vi "final_usrp_transceiver2.vi"() -> ()   [LabVIEW 2014]
uses:
  <vilib>/addons/Modulation/Analog/support/mod_Set Error Source.vi
  var_stop.vi
  <vilib>/addons/Modulation/Digital/Support/Common/Validators/mod_Generate Filter Coefficients Validate.vi
  <vilib>/addons/Modulation/Digital/General/subVIs/mod_Generate Filter Coefficients.vi
  <vilib>/measure/maspectr.llb/FFT Power Spectrum and PSD for 1 Chan (CDB).vi
  <vilib>/addons/Modulation/Digital/General/MT Apply Matched Filter (Generic).vi
  <vilib>/addons/Modulation/Digital/General/MT Align to Ideal Symbols (Generic).vi
  <instrlib>/niUSRP/niUSRP Fetch Rx Data (CDB Cluster).vi
  <instrlib>/niUSRP/niUSRP Write Tx Data (CDB Cluster).vi
  <vilib>/addons/Modulation/Digital/General/MT Apply Pulse Shaping Filter (Generic).vi
  <vilib>/addons/Modulation/niDMT.lvlib
  <vilib>/measure/NI_MAPro.lvlib
panel:
  in  "frame buffer size":i32=20
  in  "Stop":bool
  out "Frames Per Second":u32
  in  "energy threshold":dbl=-33.0 format="%#_13g"
  out "elements in frame buffer 2":i32
  out "elements in frame buffer":i32
  out "valid frames":i32
  out "elements in send buffer":i32
  in  "packet size":i32=12800
  in  "Quality (0-1000)":i32=100 caption="Quality (750)"
  out "size(s) 4":i32
  out "frame num":u32
  out "length":i32[](array[numeric])
  out "start index":i32[](array[numeric])
  out "Numeric":i32
  out "size(s) 3":i32
  out "# elements in queue 2":i32
  out "size(s) 2":i32
  out "size(s)":i32[](array[numeric])
  out "image":T1(plugin-control)
  in  "Transmit power (db)":dbl
  out "found?":bool
  out "# elements in queue":i32
  out "valid?":bool
  in  "Gray code?":bool=TRUE
  in  "Modulation":enum16{"PSK", "QAM"}(ring)
  out "packet len":u32
  in  "filter length (symbols)":i32=8
  in  "filter parameter":dbl=0.5 format="%.2f"
  in  "pulse shaping filter (none)":T2(ring)=enum."Raised Cosine"
  in  "M-PSK (4)":i32=4 caption="M-ARY"
  in  "samples per symbol (16)":i32=4
  out "packet bits length":i32
  in  "number of samples":i64=40000
  out "RX coerced gain":dbl format="%#_6f"
  out "RX coerced carrier frequency":dbl=915000000.0 format="%#_6p"
  out "RX coerced IQ rate":dbl=4000000.0 format="%#_6p"
  in  "RX active antenna":string="RX2"
  in  "RX gain":dbl format="%#_6f"
  in  "RX device names":refnum<k15>="192.168.10.2"
  out "TX coerced gain":dbl format="%#_6f"
  out "TX coerced carrier frequency":dbl=915000000.0 format="%#_6p"
  out "coerced IQ rate":dbl=4000000.0 format="%#_6p"
  in  "TX device names":refnum<k15>="192.168.10.2"
  in  "TX gain":dbl format="%#_6f"
  in  "carrier frequency":dbl=915000000.0 format="%#_6p"
  in  "IQ rate":dbl=800000.0 format="%#_6p"
  in  "stop":bool
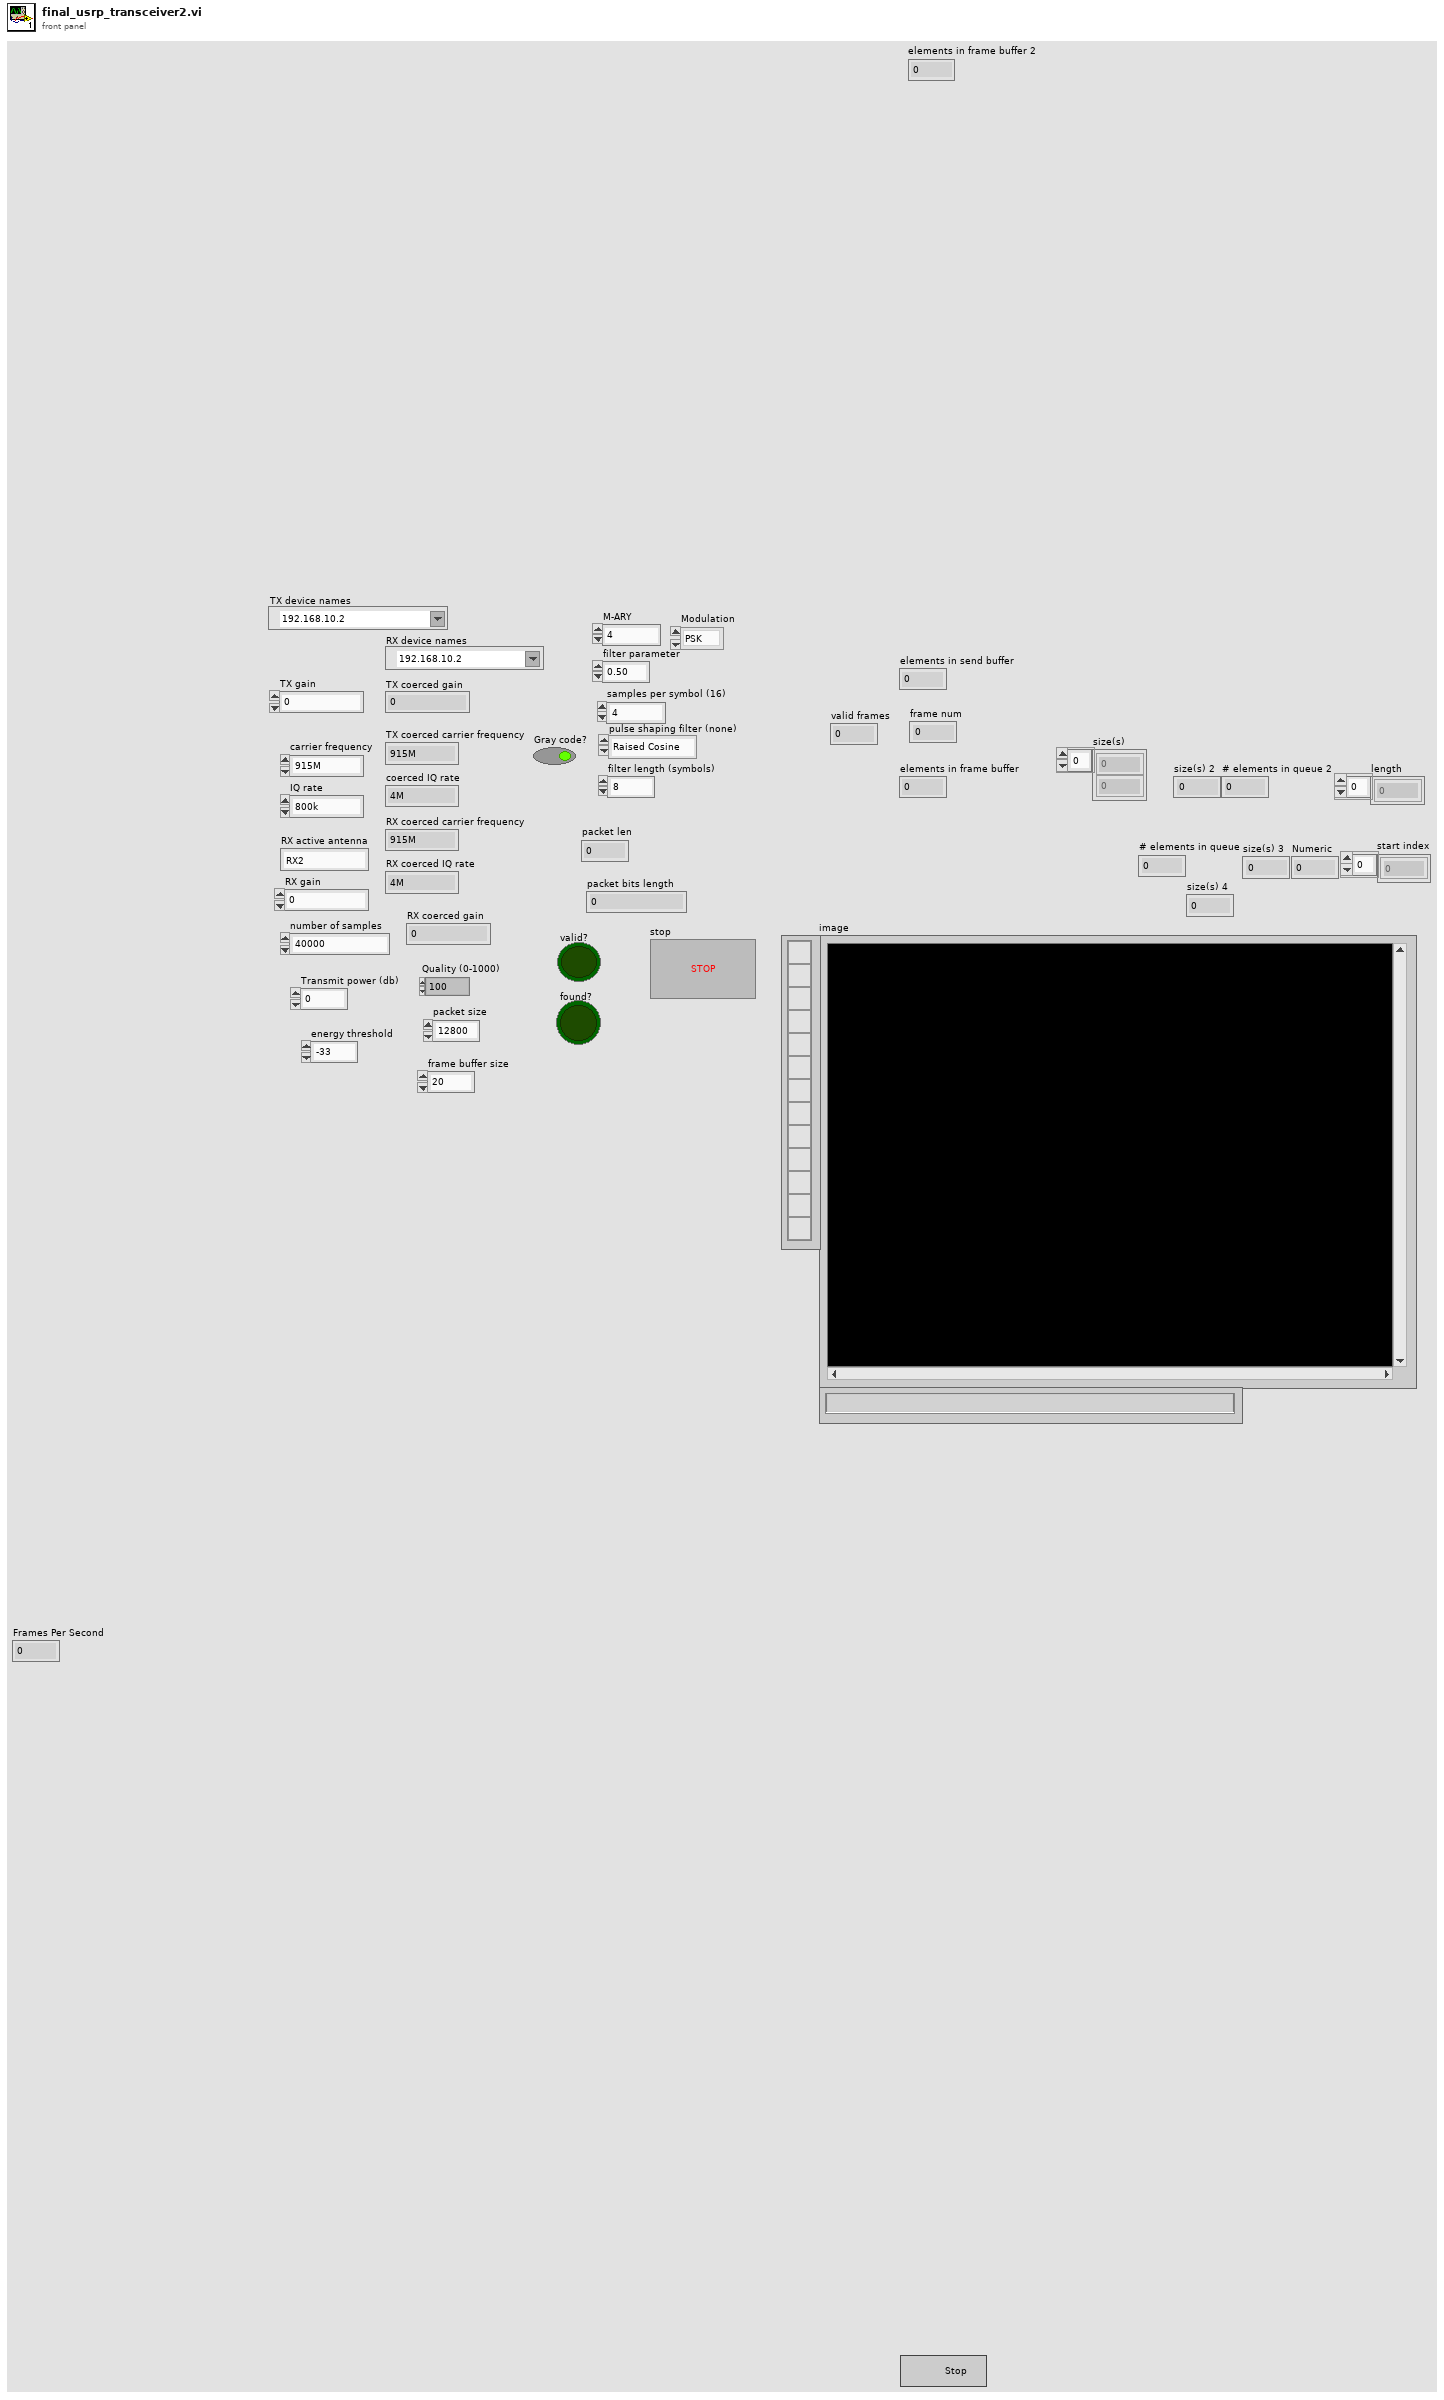
[diagram p1: front panel]
types:
  T1 = typedef "IMAQ Image.ctl" = refnum<image>
  T2 = enum16{"none", "Raised Cosine", "Root Raised Cos", "Gaussian"}
  T3 = enum16{"FSK", "PSK", "QAM", "MSK", "PAM", "ASK", "CPM"}
  T4 = cluster{"samples per symbol (16)":i32, "symbol map":cdb[], "index map":u32[]}
  T5 = cluster{"samples per symbol (16)":i32, "symbol map":cdb[], i32[]}
  T6 = typedef "IMAQ AVI2 Refnum.ctl" = refnum<k20>
  T7 = typedef "Image Type" = u32
  T8 = cluster{"Width":u32, "Height":u32, "Frames Per Second":u32, "Codec":string, "Has Data":bool}
  T9 = typedef "Semaphore RefNum" = refnum<k1>
  T10 = typedef "niAMT.lvlib/Complex Data Waveform.ctl" = cluster{"t0":dbl, "dt":dbl, "Y":cdb[]}
  T11 = typedef "imagedata.ctl" = cluster{"image type":i32, "image depth":i32, "image":u8[], "mask":u8[], "colors":u32[], "Rectangle":cluster{"left":i16, "top":i16, "right":i16, "bottom":i16}}
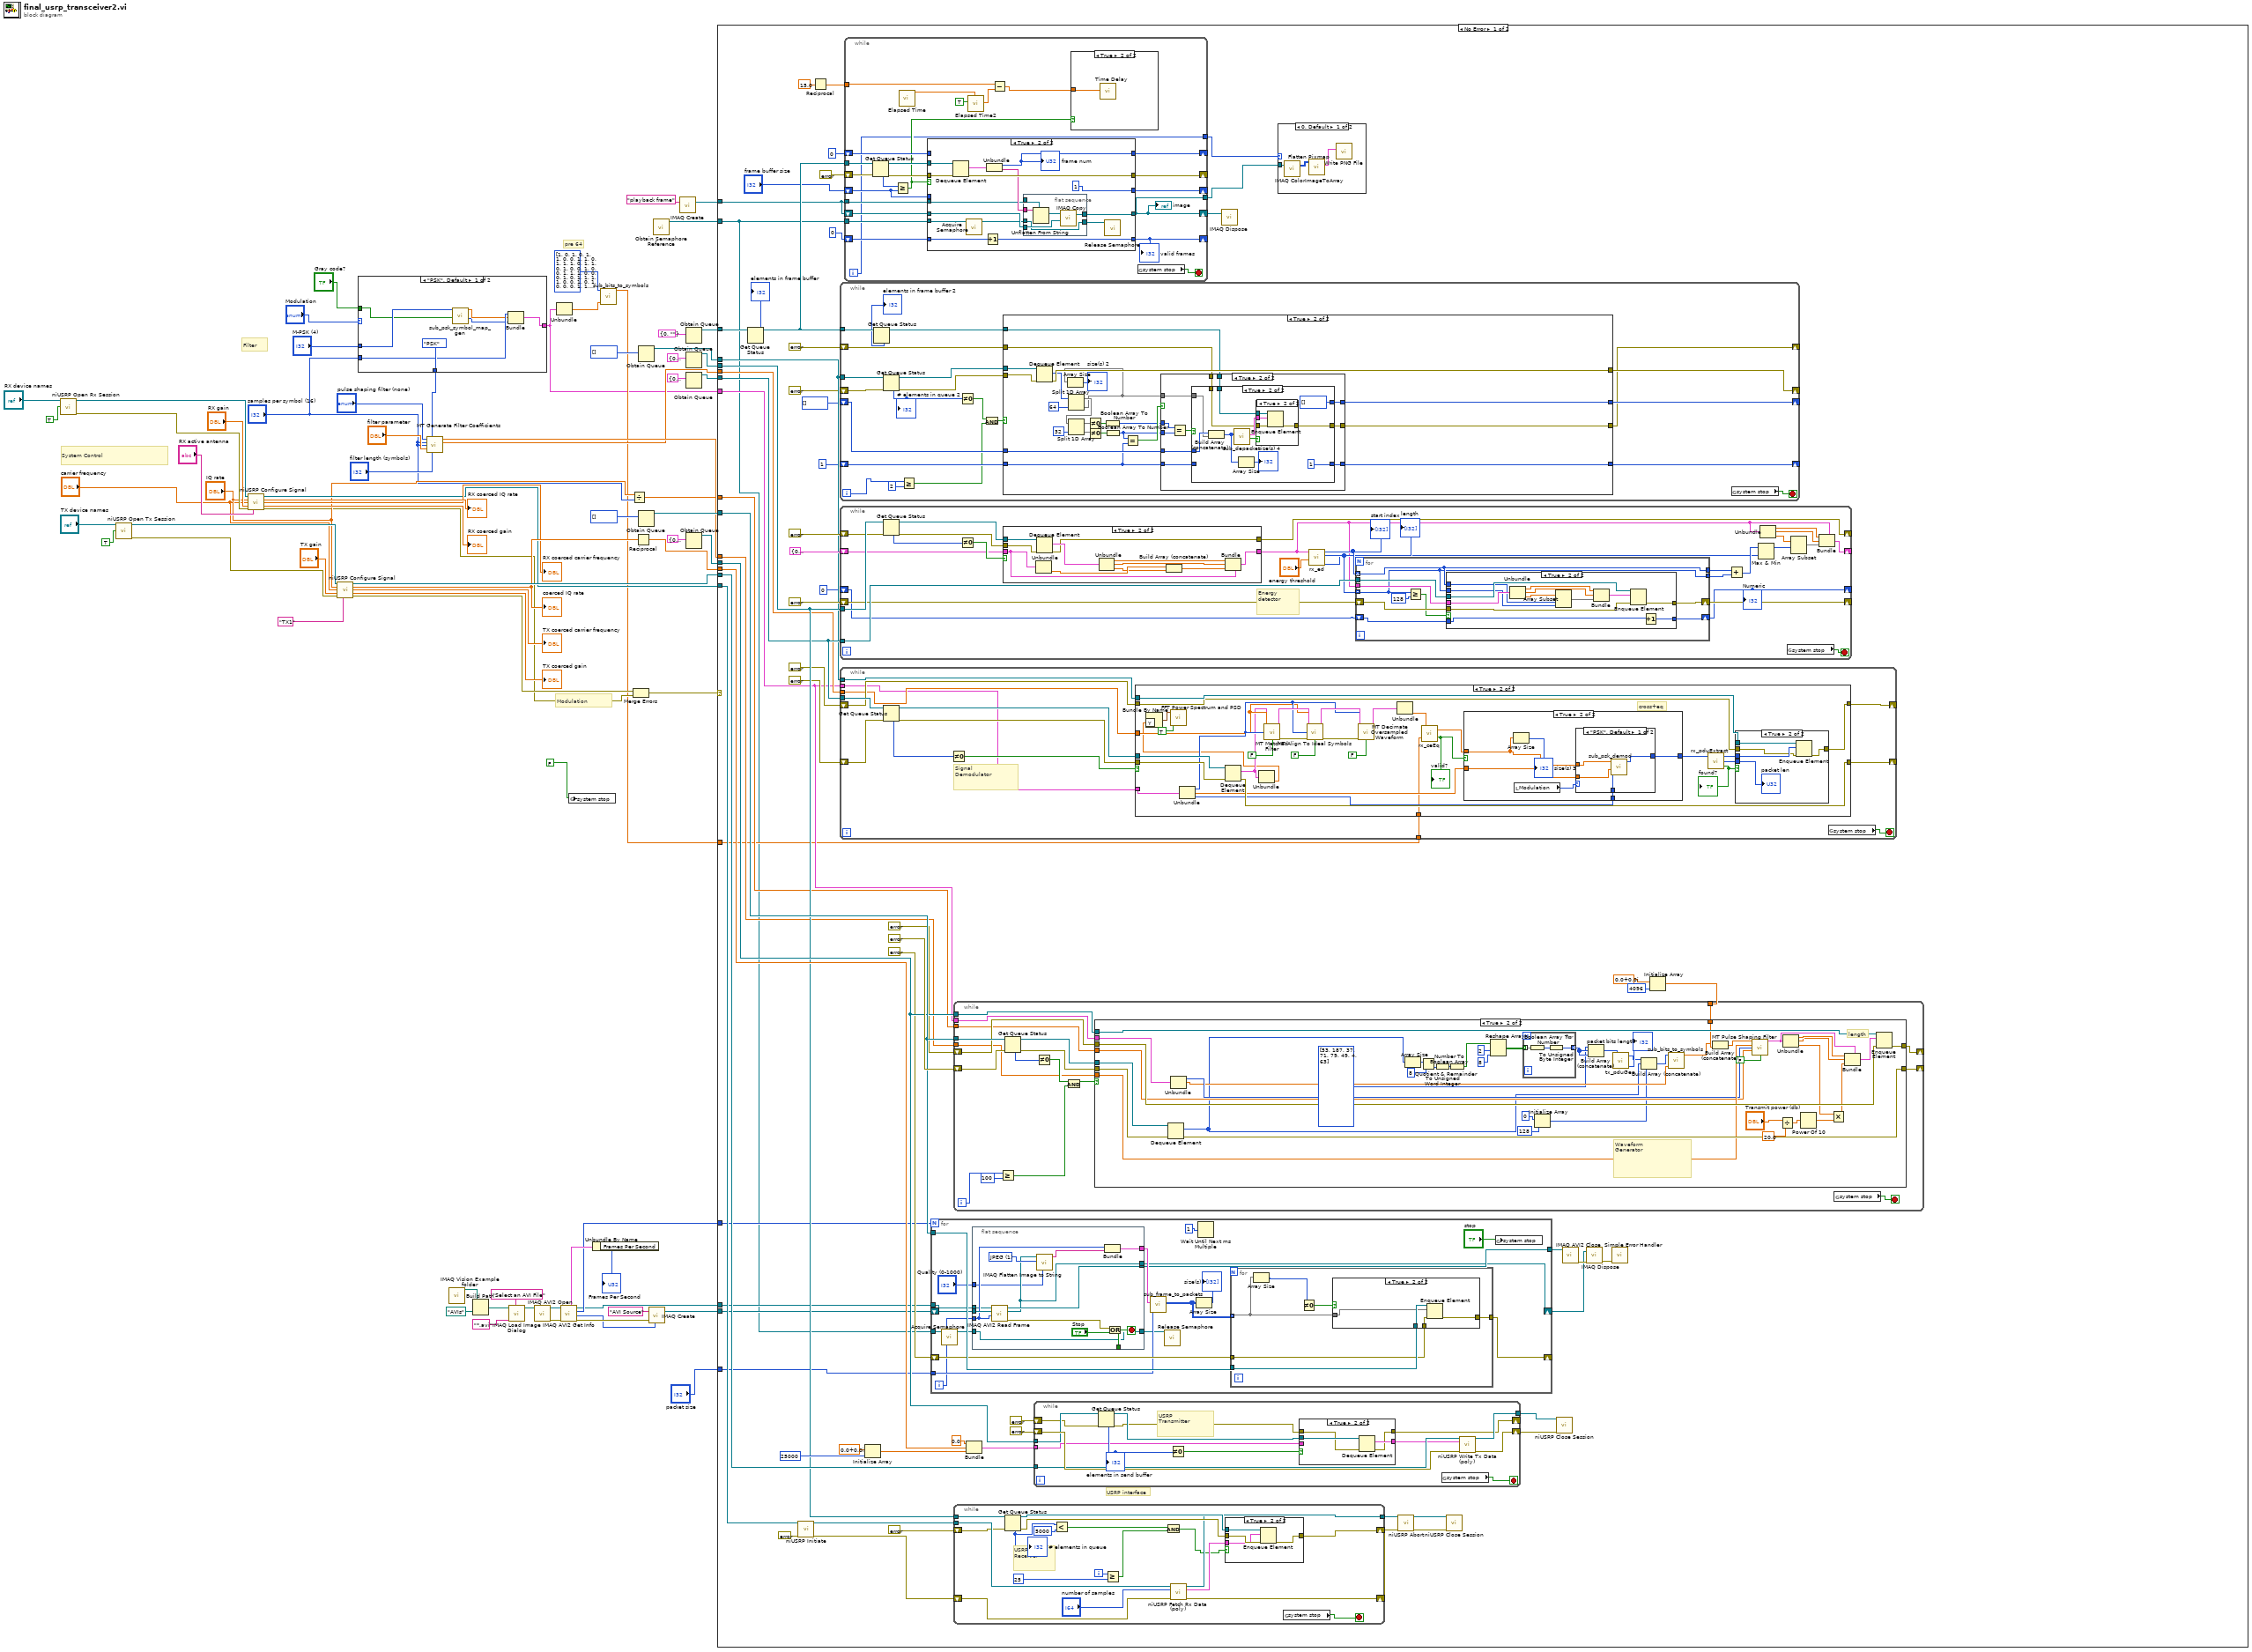
[diagram p0: block diagram]
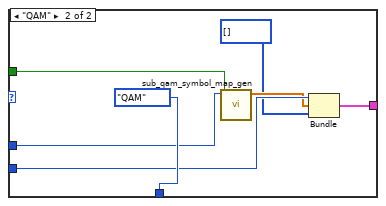
[diagram p2: hidden frame]
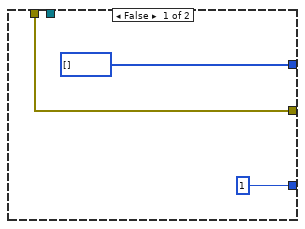
[diagram p8: hidden frame]
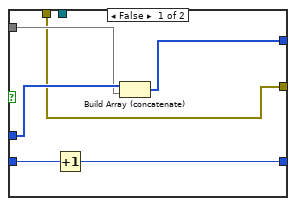
[diagram p9: hidden frame]
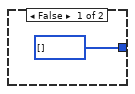
[diagram p12: hidden frame]
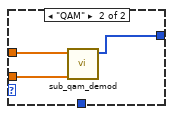
[diagram p13: hidden frame]
diagram:
  # "pre 64"
  # "Modulation"
  # "Filter"
  # "System Control"
  n1 = call <instrlib>:"niUSRP Open Rx Session.vi"("device names"="RX device names", "reset"=TRUE) -> ("session handle out"=w60:refnum<k15>, "error out"=w59:errorcluster)  [unwired: 12 in]
  n2 = call <instrlib>:"niUSRP Open Tx Session.vi"("device names"="TX device names", "reset"=TRUE) -> ("session handle out"=w73:refnum<k15>, "error out"=w72:errorcluster)  [unwired: 12 in]
  n3 = call <instrlib>:"niUSRP Configure Signal.vi"("session handle"=w60, "IQ rate"="IQ rate", "carrier frequency"="carrier frequency", "gain"="RX gain", "error in (no error)"=w59, "active antenna"="RX active antenna") -> ("session handle out"=w51:refnum<k15>, "coerced IQ rate"=→"RX coerced IQ rate":dbl, "coerced carrier frequency"=→"RX coerced carrier frequency":dbl, "coerced gain"=→"RX coerced gain":dbl, "error out"=w35:errorcluster)  [unwired: 5 in]
  n4 = call <instrlib>:"niUSRP Configure Signal.vi"("session handle"=w73, "IQ rate"="IQ rate", "carrier frequency"="carrier frequency", "gain"="TX gain", "error in (no error)"=w72, "active antenna"="TX1") -> ("session handle out"=w64:refnum<k15>, "coerced IQ rate"=w62:dbl, "coerced carrier frequency"=→"TX coerced carrier frequency":dbl, "coerced gain"=→"TX coerced gain":dbl, "error out"=w36:errorcluster)  [unwired: 5 in]
  "coerced IQ rate" <- w62
  n5 = case shown="\"PSK\", Default" "Modulation" {
    tunnel: [T3."PSK" ("modulation type") T3."QAM" ("modulation type")] -> w30
    tunnel: "M-PSK (4)" -> [w80 w86]
    tunnel: "Gray code?" -> [w79 w87]
    tunnel: "samples per symbol (16)" -> [w78 w85]
    tunnel: [w75 w82] -> w23
    frame "PSK", Default {
      n6 = call "sub_psk_symbol_map_gen.vi"("Gray code?"=w79, "M-PSK"=w80) -> ("index map"=w76:u32[], "symbol map"=w77:cdb[])  [unwired: 8 in]
      n7 = Bundle("samples per symbol (16)"=w78, "symbol map"=w77, "index map"=w76) -> (w75:T4)  [unwired: 1 in]
    }
    frame "QAM" {
      n8 = call "sub_qam_symbol_map_gen.vi"("Gray code?"=w87, "M-QAM"=w86) -> ("symbol map"=w84:cdb[])  [unwired: 9 in]
      n9 = Bundle("samples per symbol (16)"=w85, "symbol map"=w84, i32[] []) -> (w82:T5)  [unwired: 1 in]
    }
  }
  n10 = call <vilib>:"MT Generate Filter Coefficients.vi"("pulse shaping filter (none)"="pulse shaping filter (none)", "modulation type"=w30, "pulse shaping samples per symbol (16)"="samples per symbol (16)", "matched samples per symbol (16)"="samples per symbol (16)", "filter parameter"="filter parameter", "filter length (symbols)"="filter length (symbols)") -> ("pulse shaping filter coefficients"=w41:dbl[], "matched filter coefficients"=w39:dbl[])  [unwired: 7 in, 1 out]
  n11 = call "IMAQ Vision Example folder.vi"() -> ("Example Image Path"=w13:path)  [unwired: 11 in]
  n12 = Build Path(base path=w13, name or relative path=path "AVIs") -> (appended path=w10:path)
  n13 = call "IMAQ Load Image Dialog"("Prompt"="Select an AVI File" ("prompt"), "Pattern"="*.avi", "Start Path"=w10) -> ("Path"=w9:path)  [unwired: 6 in, 2 out]
  n14 = call "IMAQ AVI2 Open"("AVI File Path"=w9) -> ("error out"=w17:errorcluster, "AVI Refnum"=w16:T6)  [unwired: 2 in, 7 out]
  n15 = Unbundle(w23) -> ("symbol map"=w25:cdb[])  [unwired: 2 out]
  n16 = call "IMAQ AVI2 Get Info"("error in (no error)"=w17, "AVI Refnum"=w16) -> ("error out"=w15:errorcluster, "Image Type"=w14:T7, "Number of Frames"=w6:u32, "AVI Refnum (duplicate)"=w5:T6, "Frame Data"=w18:T8)  [unwired: 5 out]
  n17 = global write "var_stop.vi" "system stop"(FALSE) -> ()
  n18 = Unbundle By Name(w18) -> ("Frames Per Second"=→"Frames Per Second":u32)
  n19 = call "sub_bits_to_symbols.vi"("symbol map"=w25, "bits"=i16[] [1, 0, 1, 0, 1, 1, 0, 0, 1, 1, 0, 1, 1, 1, 0, 1, 1, 0, 1, 0, 0, 1, 0, 0, 1, 1, 1, 0, 0, 0, 1, 0, 1, 1, 1, 1, 0, 0, 1, 0, 1, 0, 0, 0, 1, 1, 0, 0, 0, 0, 1, 0, 0, 0, 0, 0, 1, 1, 1, 1, 1, 1, 0, 0] ("preamble(64) 2")) -> ("symbols"=w24:cdb[])  [unwired: 9 in]
  n20 = Divide(x="IQ rate", y="samples per symbol (16)") -> (x/y=w40:dbl)
  n21 = Merge Errors(w36, w35) -> (w34:errorcluster)
  n22 = Reciprocal(x=w62) -> (1/x=w61:dbl)
  n23 = Obtain Queue(element data type=i8[] [] ("output bit stream")) -> (queue out=w46:refnum<queue>)  [unwired: 4 in, 2 out]
  n24 = Obtain Queue(element data type=i16[] []) -> (queue out=w74:refnum<queue>)  [unwired: 4 in, 2 out]
  n25 = call "IMAQ Create"("Image Name"="AVI Source", "Image Type"=w14, "error in (no error)"=w15) -> ("New Image"=w4:T1)  [unwired: 1 in, 2 out]
  n26 = call <vilib>:"Obtain Semaphore Reference.vi"() -> ("semaphore"=w1:T9)  [unwired: 5 in, 2 out]
  n27 = call "IMAQ Create"("Image Name"="playback frame") -> ("New Image"=w2:T1)  [unwired: 3 in, 2 out]
  n28 = Obtain Queue(element data type=cluster{u32, "string":string} {0, "string"=""} ("frame")) -> (queue out=w21:refnum<queue>)  [unwired: 4 in, 2 out]
  n29 = Obtain Queue(element data type=cluster{"t0":dbl, "dt":dbl, "Y":cdb[]} {"t0"=0.0, "dt"=0.0, "Y"=[]} ("data")) -> (queue out=w50:refnum<queue>)  [unwired: 4 in, 2 out]
  n30 = Obtain Queue(element data type=cluster{"t0":dbl, "dt":dbl, "Y":cdb[]} {"t0"=0.0, "dt"=0.0, "Y"=[]} ("data")) -> (queue out=w47:refnum<queue>)  [unwired: 4 in, 2 out]
  n31 = Obtain Queue(element data type=cluster{"t0":dbl, "dt":dbl, "Y":cdb[]} {"t0"=0.0, "dt"=1.0, "Y"=[]} ("data")) -> (queue out=w65:refnum<queue>)  [unwired: 4 in, 2 out]
  n32 = case shown="No Error" w34 {
    tunnel: w74 -> [w155 _]
    tunnel: w65 -> [w150 _]
    tunnel: w64 -> [w151 _]
    tunnel: w61 -> [w144 _]
    tunnel: w51 -> [w139 _]
    tunnel: w50 -> [w133 _]
    tunnel: w47 -> [w129 _]
    tunnel: w46 -> [w127 _]
    tunnel: w23 -> [w121 _]
    tunnel: w41 -> [w124 _]
    tunnel: w40 -> [w123 _]
    tunnel: w39 -> [w122 _]
    tunnel: w24 -> [w115 _]
    tunnel: w21 -> [w111 _]
    tunnel: "packet size" -> [w105 _]
    tunnel: w6 -> [w100 _]
    tunnel: w5 -> [w99 _]
    tunnel: w4 -> [w98 _]
    tunnel: w2 -> [w92 _]
    tunnel: w1 -> [w91 _]
    frame No Error {
      # "USRP interface"
      n33 = Get Queue Status(queue=w111) -> (queue out=w103:refnum<queue>, # elements in queue=→"elements in frame buffer":i32)  [unwired: 2 in, 6 out]
      n34 = call <instrlib>:"niUSRP Initiate.vi"("session handle"=w139, "error in (no error)"=errorcluster {"status"=FALSE, "code"=0, "source"=""}) -> ("session handle out"=w138:refnum<k15>, "error out"=w137:errorcluster)  [unwired: 12 in]
      n35 = Reciprocal(x=15.0) -> (1/x=w106:dbl)
      n36 = while {
        tunnel: w127 -> [w274]
        shift-right: [w267] -> _
        shift-left: errorcluster {"status"=FALSE, "code"=0, "source"=""} ("error out") -> [w273]
        shift-right: [w265] -> _
        shift-left: u32 1 -> [w266]
        shift-right: [w264] -> _
        shift-left: i8[] [] ("second subarray") -> [w263]
        tunnel: w103 -> [w262]
        shift-right: [w260] -> _
        shift-left: errorcluster {"status"=FALSE, "code"=0, "source"=""} ("error out") -> [w261]
        i -> [w258]
        stop <- w272 stop-if-true
        n37 = Get Queue Status(queue=w262) -> (queue out=w255:refnum<queue>, # elements in queue=→"elements in frame buffer 2":i32)  [unwired: 2 in, 6 out]
        n38 = Get Queue Status(queue=w274, error in (no error)=w273) -> (queue out=w269:refnum<queue>, error out=w268:errorcluster, # elements in queue=w271:i32)  [unwired: 1 in, 5 out]
        "# elements in queue 2" <- w271
        n39 = Greater Or Equal?(x=w258, y=2) -> (x >= y?=w257:bool)
        n40 = Not Equal To 0?(x=w271) -> (x != 0?=w270:bool)
        n41 = And(x=w270, y=w257) -> (x .and. y?=w256:bool)
        n42 = case shown="True" w256 {
          tunnel: w269 -> [_ w301]
          tunnel: w268 -> [w278 w300]
          tunnel: [w278 w299] -> w267
          tunnel: w266 -> [w277 w285]
          tunnel: [w277 w286] -> w265
          tunnel: [w275 w290] -> w264
          tunnel: w263 -> [w275 w287]
          tunnel: w255 -> [_ w284]
          tunnel: w261 -> [w276 w283]
          tunnel: [w276 w282] -> w260
          frame False {
          }
          frame True {
            n43 = Dequeue Element(queue=w301, error in (no error)=w300) -> (element=w281:i8[], error out=w299:errorcluster)  [unwired: 1 in, 2 out]
            n44 = Split 1D Array(array=w281, index=64) -> (first subarray=w292:i8[], second subarray=w279:i8[])
            n45 = Array Size(array=w279) -> (size(s)=→"size(s) 2":i32)
            n46 = Split 1D Array(array=w292, index=32) -> (first subarray=w295:i8[], second subarray=w296:i8[])
            n47 = Not Equal To 0?(x=w295) -> (x != 0?=w294:bool[])
            n48 = Not Equal To 0?(x=w296) -> (x != 0?=w293:bool[])
            n49 = Boolean Array To Number(Boolean array=w294) -> (number=w289:u32)
            n50 = Boolean Array To Number(Boolean array=w293) -> (number=w288:u32)
            n51 = Equal?(x=w288, y=w285) -> (x = y?=w291:bool)
            n52 = case shown="True" w291 {
              tunnel: [i8[] [] ("second subarray") w312] -> w290
              tunnel: w289 -> [_ w315]
              tunnel: w288 -> [_ w314]
              tunnel: w287 -> [_ w311]
              tunnel: w279 -> [_ w310]
              tunnel: [u32 1 w309] -> w286
              tunnel: w285 -> [_ w308]
              tunnel: w284 -> [_ w307]
              tunnel: w283 -> [w302 w306]
              tunnel: [w302 w305] -> w282
              frame False {
              }
              frame True {
                n53 = Equal?(x=w315, y=w314) -> (x = y?=w313:bool)
                n54 = case shown="True" w313 {
                  tunnel: [w319 i8[] [] ("second subarray")] -> w312
                  tunnel: w311 -> [w321 w330]
                  tunnel: w310 -> [w320 w329]
                  tunnel: [w317 u32 1] -> w309
                  tunnel: w308 -> [w318 _]
                  tunnel: w307 -> [_ w328]
                  tunnel: w306 -> [w316 w326]
                  tunnel: [w316 w325] -> w305
                  frame False {
                    n55 = Increment(x=w318) -> (x+1=w317:u32)
                    n56 = Build Array (concatenate)(w321, w320) -> (w319:i8[])
                  }
                  frame True {
                    n57 = Build Array (concatenate)(w330, w329) -> (w324:i8[])
                    n58 = call "sub_depacket.vi"("bitstream"=w324) -> ("CRC valid"=w322:bool, "frame"=w327:cluster{u32, "string":string})  [unwired: 9 in]
                    n59 = Array Size(array=w324) -> (size(s)=→"size(s) 4":i32)
                    n60 = case shown="True" w322 {
                      tunnel: w328 -> [_ w337]
                      tunnel: w327 -> [_ w336]
                      tunnel: w326 -> [w333 w335]
                      tunnel: [w333 w334] -> w325
                      frame False {
                      }
                      frame True {
                        n61 = Enqueue Element(queue=w337, element=w336, error in (no error)=w335) -> (error out=w334:errorcluster)  [unwired: 1 in, 2 out]
                      }
                    }
                  }
                }
              }
            }
          }
        }
        n62 = global read "var_stop.vi" "system stop"() -> (w272:bool)
      }
      n63 = while {
        tunnel: w133 -> [w432]
        shift-right: [w425] -> _
        shift-left: errorcluster {"status"=FALSE, "code"=0, "source"=""} ("error out") -> [w431]
        shift-right: [w411] -> _
        shift-left: cluster{"t0":dbl, "dt":dbl, "Y":cdb[]} {"t0"=0.0, "dt"=0.0, "Y"=[]} ("data") -> [w426]
        tunnel: w129 -> [w424]
        shift-right: [w423] -> _
        shift-left: errorcluster {"status"=FALSE, "code"=0, "source"=""} ("error out") -> [w422]
        shift-right: [w406] -> _
        shift-left: 0 -> [w407]
        stop <- w421 stop-if-true
        # "Energy\ndetector"
        n64 = Get Queue Status(queue=w432, error in (no error)=w431) -> (queue out=w427:refnum<queue>, error out=w428:errorcluster, # elements in queue=w430:i32)  [unwired: 1 in, 5 out]
        n65 = Not Equal To 0?(x=w430) -> (x != 0?=w429:bool)
        n66 = case shown="True" w429 {
          tunnel: w428 -> [w459 w470]
          tunnel: w427 -> [_ w469]
          tunnel: w426 -> [w458 w464]
          tunnel: [w459 w461] -> w425
          tunnel: [w458 w460] -> w418
          frame False {
          }
          frame True {
            n67 = Unbundle(w464) -> ("Y"=w467:cdb[])  [unwired: 2 out]
            n68 = Dequeue Element(queue=w469, error in (no error)=w470) -> (element=w468:cluster{"t0":dbl, "dt":dbl, "Y":cdb[]}, error out=w461:errorcluster)  [unwired: 1 in, 2 out]
            n69 = Unbundle(w468) -> ("t0"=w463:dbl, "dt"=w462:dbl, "Y"=w466:cdb[])
            n70 = Build Array (concatenate)(w467, w466) -> (w465:cdb[])
            n71 = Bundle(cluster=w464, "t0"=w463, "dt"=w462, "Y"=w465) -> (w460:cluster{"t0":dbl, "dt":dbl, "Y":cdb[]})
          }
        }
        n72 = call "rx_ed.vi"("energy threshold"="energy threshold", "Wavefrom"=w418) -> ("first pulse"=w408:i32, "length"=w419:i32[], "start index"=w420:i32[])  [unwired: 7 in]
        "start index" <- w420
        "length" <- w419
        n73 = for {
          tunnel: w424 -> [w442]
          tunnel: w418 -> [w439]
          shift-right: [w441] -> w423
          shift-left: w422 -> [w440]
          tunnel: w420 -> [w438] mode=indexing
          tunnel: w419 -> [w437] mode=indexing
          tunnel: [w438] -> w414
          tunnel: [w437] -> w413
          shift-right: [w433] -> w406
          shift-left: w407 -> [w434]
          n74 = Greater Or Equal?(x=w437, y=128) -> (x >= y?=w435:bool)
          n75 = case shown="True" w435 {
            tunnel: w442 -> [_ w457]
            tunnel: [w444 w456] -> w441
            tunnel: w440 -> [w444 w455]
            tunnel: w439 -> [_ w454]
            tunnel: w438 -> [_ w448]
            tunnel: w437 -> [_ w447]
            tunnel: w434 -> [w443 w446]
            tunnel: [w443 w445] -> w433
            frame False {
            }
            frame True {
              n76 = Unbundle(w454) -> ("t0"=w452:dbl, "dt"=w453:dbl, "Y"=w450:cdb[])
              n77 = Array Subset(array=w450, index=w448, length=w447) -> (w449:cdb[])
              n78 = Bundle("t0"=w452, "dt"=w453, w449) -> (w451:cluster{"t0":dbl, "dt":dbl, cdb[]})  [unwired: 1 in]
              n79 = Enqueue Element(queue=w457, element=w451, error in (no error)=w455) -> (error out=w456:errorcluster)  [unwired: 1 in, 2 out]
              n80 = Increment(x=w446) -> (x+1=w445:i32)
            }
          }
        }
        "Numeric" <- w406
        n81 = Add(x=w414, y=w413) -> (x+y=w410:i32)
        n82 = Max & Min(x=w410, y=w408) -> (max(x,y)=w409:i32)  [unwired: 1 out]
        n83 = Unbundle(w418) -> ("t0"=w417:dbl, "dt"=w416:dbl, "Y"=w415:cdb[])
        n84 = global read "var_stop.vi" "system stop"() -> (w421:bool)
        n85 = Array Subset(array=w415, index=w409) -> (w412:cdb[])  [unwired: 1 in]
        n86 = Bundle(cluster=w418, "t0"=w417, "dt"=w416, "Y"=w412) -> (w411:cluster{"t0":dbl, "dt":dbl, "Y":cdb[]})
      }
      n87 = while {
        tunnel: w129 -> [w351]
        shift-right: [w345] -> _
        shift-left: errorcluster {"status"=FALSE, "code"=0, "source"=""} ("error out") -> [w350]
        tunnel: w127 -> [w344]
        shift-right: [w343] -> _
        shift-left: errorcluster {"status"=FALSE, "code"=0, "source"=""} ("error out") -> [w342]
        tunnel: w122 -> [w340]
        tunnel: w121 -> [w339]
        tunnel: w115 -> [w338]
        stop <- w341 stop-if-true
        # "Signal \nDemodulator"
        n88 = Get Queue Status(queue=w351, error in (no error)=w350) -> (queue out=w347:refnum<queue>, error out=w346:errorcluster, # elements in queue=w349:i32)  [unwired: 1 in, 5 out]
        n89 = Not Equal To 0?(x=w349) -> (x != 0?=w348:bool)
        n90 = case shown="True" w348 {
          tunnel: w347 -> [_ w383]
          tunnel: w346 -> [w353 w384]
          tunnel: [w353 w382] -> w345
          tunnel: w344 -> [_ w372]
          tunnel: [w352 w371] -> w343
          tunnel: w342 -> [w352 w370]
          tunnel: w340 -> [_ w359]
          tunnel: w339 -> [_ w363]
          tunnel: w338 -> [_ w356]
          frame False {
          }
          frame True {
            # "cross+eq"
            n91 = Unbundle(w363) -> ("samples per symbol (16)"=w362:i32, "symbol map"=w361:cdb[], "index map"=w360:u32[])
            n92 = Dequeue Element(queue=w383, error in (no error)=w384) -> (element=w355:cluster{"t0":dbl, "dt":dbl, "Y":cdb[]}, error out=w382:errorcluster)  [unwired: 1 in, 2 out]
            n93 = Unbundle(w355) -> ("Y"=w354:cdb[])  [unwired: 2 out]
            n94 = Bundle By Name("Y"=w354) -> (w358:waveform(cdb))  [unwired: 1 in]
            n95 = call-poly <vilib>:"FFT Power Spectrum and PSD.vi"("dB On (F)"=TRUE, "time signal"=w358) -> ()  [unwired: 6 in, 4 out]
            n96 = call-poly <vilib>:"MT Matched Filter.vi"("input complex waveform"=w355, "matched filter coefficients"=w359, "samples per symbol (16)"=w362, "reset? (T)"=FALSE) -> ("output complex waveform"=w381:T10, "error out"=w380:errorcluster)  [unwired: 10 in]
            n97 = call-poly <vilib>:"MT Align To Ideal Symbols.vi"("input complex waveform"=w381, "matched filter coefficients"=w359, "samples per symbol (16)"=w362, "error in (no error)"=w380, "reset? (T)"=FALSE) -> ("output complex waveform"=w378:T10, "error out"=w379:errorcluster)  [unwired: 8 in, 1 out]
            n98 = call <vilib>:"MT Decimate Oversampled Waveform.vi"("input complex waveform"=w378, "decimation factor"=w362, "error in (no error)"=w379, "reset? (T)"=FALSE) -> ("output complex waveform"=w377:T10)  [unwired: 10 in, 1 out]
            n99 = Unbundle(w377) -> ("Y"=w373:cdb[])  [unwired: 2 out]
            n100 = call "rx_ceEq.vi"("preamble"=w356, "symbols"=w373) -> ("valid?"=w368:bool, "eq symbols"=w369:cdb[])
            "valid?" <- w368
            n101 = case shown="True" w368 {
              tunnel: [i8[] [] ("output bit stream") w389] -> w376
              tunnel: w361 -> [_ w390]
              tunnel: w369 -> [_ w387]
              tunnel: w360 -> [_ w388]
              frame False {
              }
              frame True {
                n102 = Array Size(array=w387) -> (size(s)=→"size(s) 3":i32)
                n103 = local read "Modulation"() -> (w391:enum16{"PSK", "QAM"})
                n104 = case shown="\"PSK\", Default" w391 {
                  tunnel: w387 -> [w395 w398]
                  tunnel: w390 -> [w394 w397]
                  tunnel: [w392 w396] -> w389
                  tunnel: w388 -> [w393 _]
                  frame "PSK", Default {
                    n105 = call "sub_psk_demod.vi"("index map"=w393, "symbol map"=w394, "symbol"=w395) -> ("bitstream"=w392:i16[])  [unwired: 8 in]
                  }
                  frame "QAM" {
                    n106 = call "sub_qam_demod.vi"("symbol map"=w397, "symbol"=w398) -> ("bitstream"=w396:i16[])  [unwired: 9 in]
                  }
                }
              }
            }
            n107 = call "rx_pduExtract.vi"("output bit stream"=w376) -> ("found?"=w375:bool, "packet len"=w367:u32, "ppdu"=w374:i8[])  [unwired: 2 in]
            "found?" <- w375
            n108 = case shown="True" w375 {
              tunnel: w374 -> [_ w402]
              tunnel: w372 -> [_ w404]
              tunnel: [w399 w403] -> w371
              tunnel: w370 -> [w399 w400]
              tunnel: w367 -> [_ w401]
              frame False {
              }
              frame True {
                n109 = Enqueue Element(queue=w404, element=w402, error in (no error)=w400) -> (error out=w403:errorcluster)  [unwired: 1 in, 2 out]
                "packet len" <- w401
              }
            }
          }
        }
        n110 = global read "var_stop.vi" "system stop"() -> (w341:bool)
      }
      n111 = while {
        tunnel: w103 -> [w226]
        shift-right: [w222] -> _
        shift-left: errorcluster {"status"=FALSE, "code"=0, "source"=""} ("error out") -> [w225]
        shift-right: [w219] -> _
        shift-left: 0 -> [w218]
        tunnel: w106 -> [w214]
        shift-right: [w215] -> _
        shift-left: 0 -> [w216]
        shift-right: [w210] -> _
        shift-left: "frame buffer size" -> [w209]
        shift-right: [w203] -> w93
        shift-left: w92 -> [w207]
        tunnel: w92 -> [w206]
        tunnel: w91 -> [w205]
        tunnel: [w204] -> w90
        tunnel: [w203] -> w89
        i -> [w204]
        stop <- w221 stop-if-true
        n112 = Get Queue Status(queue=w226, error in (no error)=w225) -> (queue out=w224:refnum<queue>, error out=w223:errorcluster, # elements in queue=w211:i32)  [unwired: 1 in, 5 out]
        n113 = Greater Or Equal?(x=w211, y=w209) -> (x >= y?=w208:bool)
        n114 = call "Elapsed Time"() -> ("Present (s)"=w213:dbl)  [unwired: 12 in, 7 out]
        n115 = case shown="True" w208 {
          tunnel: w224 -> [_ w247]
          tunnel: w223 -> [w232 w246]
          tunnel: [w232 w244] -> w222
          tunnel: [w231 w242] -> w219
          tunnel: w218 -> [w231 _]
          tunnel: w216 -> [w230 w241]
          tunnel: [w230 w240] -> w215
          tunnel: [w229 1] -> w210
          tunnel: w209 -> [w229 _]
          tunnel: [w228 w237] -> w203
          tunnel: w207 -> [w228 w236]
          tunnel: w206 -> [_ w238]
          tunnel: w205 -> [_ w235]
          frame False {
          }
          frame True {
            n116 = Dequeue Element(queue=w247, error in (no error)=w246) -> (element=w245:cluster{u32, "string":string}, error out=w244:errorcluster)  [unwired: 1 in, 2 out]
            n117 = call <vilib>:"Acquire Semaphore.vi"("semaphore"=w235) -> ("semaphore out"=w234:T9)  [unwired: 4 in, 2 out]
            n118 = Increment(x=w241) -> (x+1=w240:i32)
            n119 = Unbundle(w245) -> (w242:u32, "string"=w243:string)
            "frame num" <- w242
            n120 = flat-sequence {
              tunnel: w243 -> [w253]
              tunnel: w238 -> [w252]
              tunnel: [w250] -> w237
              tunnel: w236 -> [w249]
              tunnel: w234 -> [w248]
              tunnel: [w248] -> w233
              frame #0 {
                n121 = Unflatten From String(type=w252, binary string=w253) -> (value=w251:T1)  [unwired: 3 in, 2 out]
                n122 = call "IMAQ Copy"("Image Dst"=w249, "Image Src"=w251) -> ("Image Dst Out"=w250:T1)  [unwired: 4 in, 1 out]
              }
            }
            n123 = call <vilib>:"Release Semaphore.vi"("semaphore"=w233) -> ()  [unwired: 5 in, 2 out]
          }
        }
        "valid frames" <- w215
        "image" <- w203
        n124 = call "Elapsed Time2"("Reset"=TRUE, "Set Start Time (s)"=w213) -> ("Elapsed Time (s)"=w217:dbl)  [unwired: 10 in, 7 out]
        n125 = Subtract(x=w214, y=w217) -> (x-y=w212:dbl)
        n126 = case shown="True" w208 {
          tunnel: w212 -> [_ w227]
          frame False {
          }
          frame True {
            n127 = call "Time Delay"("Delay Time (s)"=w227) -> ()  [unwired: 10 in, 1 out]
          }
        }
        n128 = global read "var_stop.vi" "system stop"() -> (w221:bool)
      }
      n129 = Initialize Array(cdb 0.0+0.0i, 25000 ("dimension size")) -> (w145:cdb[])
      n130 = for {
        N: w100 -> [_]
        tunnel: w155 -> [w177]
        shift-right: [w175] -> _
        shift-left: errorcluster {"status"=FALSE, "code"=0, "source"=""} ("error out") -> [w176]
        tunnel: w105 -> [w171]
        tunnel: w99 -> [w167]
        tunnel: [w166] -> w95
        shift-right: [w165] -> w94
        shift-left: w98 -> [w170]
        tunnel: w91 -> [w162]
        i -> [w169]
        stop <- w164 stop-if-true
        n131 = call <vilib>:"Acquire Semaphore.vi"("semaphore"=w162) -> ("semaphore out"=w161:T9)  [unwired: 4 in, 2 out]
        n132 = flat-sequence {
          tunnel: w170 -> [w187]
          tunnel: w169 -> [w186]
          tunnel: [w185] -> w168
          tunnel: w167 -> [w184]
          tunnel: [w183] -> w166
          tunnel: [w182] -> w165
          tunnel: [w181] -> w164
          tunnel: "Quality (0-1000)" -> [w180]
          tunnel: w161 -> [w179]
          tunnel: [w179] -> w160
          frame #0 {
            w189 = 1 items=["None", "JPEG", "PACKED BINARY"] ("Compression (None)")
            n133 = call "IMAQ AVI2 Read Frame"("Frame Number"=w186, "Image"=w187, "AVI Refnum"=w184) -> ("error out"=w190:errorcluster, "Image Out"=w182:T1, "AVI Refnum (duplicate)"=w183:T6)  [unwired: 1 in, 5 out]
            n134 = call "IMAQ Flatten Image to String"("Quality (750)"=w180, "Compression (None)"=w189, "Image"=w182) -> ("Data String"=w188:string)  [unwired: 7 in, 1 out]
            n135 = Bundle(w186, "Data String"=w188) -> (w185:cluster{i32, "Data String":string})  [unwired: 1 in]
            n136 = Or(x=w190, y="Stop") -> (x .or. y?=w181:bool)
          }
        }
        n137 = call "sub_frame_to_packets.vi"("packet size"=w171, "Cluster"=w168) -> ("packets"=w174:i16[][])  [unwired: 9 in]
        n138 = call <vilib>:"Release Semaphore.vi"("semaphore"=w160) -> ()  [unwired: 5 in, 2 out]
        n139 = Array Size(array=w174) -> (size(s)=→"size(s)":i32[])
        n140 = Wait Until Next ms Multiple(millisecond multiple=u32 1) -> ()  [unwired: 1 out]
        n141 = for {
          tunnel: w177 -> [w197]
          tunnel: w176 -> [w196]
          tunnel: [w195] -> w175
          tunnel: w174 -> [w192] mode=indexing
          n142 = Array Size(array=w192) -> (size(s)=w193:i32)
          n143 = Not Equal To 0?(x=w193) -> (x != 0?=w194:bool)
          n144 = case shown="True" w194 {
            tunnel: w192 -> [_ w199]
            tunnel: w197 -> [_ w202]
            tunnel: w196 -> [w198 w201]
            tunnel: [w198 w200] -> w195
            frame False {
            }
            frame True {
              n145 = Enqueue Element(queue=w202, element=w199, error in (no error)=w201) -> (error out=w200:errorcluster)  [unwired: 1 in, 2 out]
            }
          }
        }
        n146 = global write "var_stop.vi" "system stop"("stop") -> ()
      }
      n147 = while {
        tunnel: w138 -> [w489]
        shift-right: [w478] -> w134
        shift-left: w137 -> [w488]
        tunnel: w133 -> [w486]
        shift-right: [w480] -> _
        shift-left: errorcluster {"status"=FALSE, "code"=0, "source"=""} ("error out") -> [w485]
        tunnel: [w479] -> w135
        i -> [w476]
        stop <- w477 stop-if-true
        # "USRP\nReceiver"
        n148 = Get Queue Status(queue=w486, error in (no error)=w485) -> (queue out=w482:refnum<queue>, error out=w481:errorcluster, # elements in queue=w484:i32)  [unwired: 1 in, 5 out]
        "# elements in queue" <- w484
        n149 = Less?(x=w484, y=5000) -> (x < y?=w474:bool)
        n150 = Greater Or Equal?(x=w476, y=25) -> (x >= y?=w473:bool)
        n151 = And(x=w474, y=w473) -> (x .and. y?=w471:bool)
        n152 = call-poly <instrlib>:"niUSRP Fetch Rx Data (poly).vi"("session handle"=w489, "number of samples"="number of samples", "error in (no error)"=w488) -> ("session handle out"=w479:refnum<k15>, "data"=w472:cluster{"t0":dbl, "dt":dbl, "Y":cdb[]}, "error out"=w478:errorcluster)  [unwired: 9 in, 1 out]
        n153 = case shown="True" w471 {
          tunnel: w482 -> [_ w494]
          tunnel: w481 -> [w490 w493]
          tunnel: [w490 w492] -> w480
          tunnel: w472 -> [_ w491]
          frame False {
          }
          frame True {
            n154 = Enqueue Element(queue=w494, element=w491, error in (no error)=w493) -> (error out=w492:errorcluster)  [unwired: 1 in, 2 out]
          }
        }
        n155 = global read "var_stop.vi" "system stop"() -> (w477:bool)
      }
      n156 = Bundle(0.0, w144, w145) -> (w142:cluster{dbl, dbl, cdb[]})  [unwired: 1 in]
      n157 = while {
        shift-right: [w504] -> w154
        shift-left: errorcluster {"status"=FALSE, "code"=0, "source"=""} ("error out") -> [w502]
        tunnel: [w503] -> w153
        tunnel: w151 -> [w501]
        tunnel: w150 -> [w499]
        shift-right: [w497] -> _
        shift-left: errorcluster {"status"=FALSE, "code"=0, "source"=""} ("error out") -> [w498]
        tunnel: w142 -> [w496]
        stop <- w495 stop-if-true
        # "USRP\nTransmitter"
        n158 = Get Queue Status(queue=w499, error in (no error)=w498) -> (queue out=w506:refnum<queue>, error out=w505:errorcluster, # elements in queue=w508:i32)  [unwired: 1 in, 5 out]
        "elements in send buffer" <- w508
        n159 = Not Equal To 0?(x=w508) -> (x != 0?=w507:bool)
        n160 = case shown="True" w507 {
          tunnel: w506 -> [_ w514]
          tunnel: w505 -> [w509 w513]
          tunnel: [w510 w512] -> w500
          tunnel: [w509 w511] -> w497
          tunnel: w496 -> [w510 _]
          frame False {
          }
          frame True {
            n161 = Dequeue Element(queue=w514, error in (no error)=w513) -> (element=w512:cluster{"t0":dbl, "dt":dbl, "Y":cdb[]}, error out=w511:errorcluster)  [unwired: 1 in, 2 out]
          }
        }
        n162 = global read "var_stop.vi" "system stop"() -> (w495:bool)
        n163 = call-poly <instrlib>:"niUSRP Write Tx Data (poly).vi"("session handle"=w501, "data"=w500, "error in (no error)"=w502) -> ("session handle out"=w503:refnum<k15>, "error out"=w504:errorcluster)  [unwired: 11 in]
      }
      n164 = call "IMAQ Dispose"("Image"=w93) -> ()  [unwired: 2 in, 4 out]
      n165 = case shown="0, Default" w90 {
        tunnel: w89 -> [w159 _]
        frame 0, Default {
          n166 = call "IMAQ ColorImageToArray"("Image"=w159) -> ("Image Pixels (U32)"=w158:u32[][])  [unwired: 3 in, 2 out]
          n167 = call <vilib>:"Flatten Pixmap.vi"("24-bit pixmap"=w158) -> ("image data"=w157:T11)  [unwired: 10 in]
          n168 = call <vilib>:"Write PNG File.vi"("image data"=w157) -> ()  [unwired: 9 in, 2 out]
        }
        frame 1 {
        }
      }
      n169 = call <instrlib>:"niUSRP Abort.vi"("session handle"=w135, "error in (no error)"=w134) -> ("session handle out"=w141:refnum<k15>, "error out"=w140:errorcluster)  [unwired: 12 in]
      n170 = call <instrlib>:"niUSRP Close Session.vi"("session handle"=w141, "error in (no error)"=w140) -> ()  [unwired: 13 in, 1 out]
      n171 = call <instrlib>:"niUSRP Close Session.vi"("session handle"=w153, "error in (no error)"=w154) -> ()  [unwired: 13 in, 1 out]
      n172 = call "IMAQ AVI2 Close"("AVI Refnum"=w95) -> ("error out"=w96:errorcluster)  [unwired: 1 in, 9 out]
      n173 = call "IMAQ Dispose"("Image"=w94, "error in (no error)"=w96) -> ("error out"=w97:errorcluster)  [unwired: 1 in, 3 out]
      n174 = call <vilib>:"Simple Error Handler.vi"("error in (no error)"=w97) -> ()  [unwired: 1 in, 8 out]
      n175 = Initialize Array(cdb 0.0+0.0i, 4096 ("dimension size")) -> (w116:cdb[])
      n176 = while {
        tunnel: w155 -> [w530]
        shift-right: [w527] -> _
        shift-left: errorcluster {"status"=FALSE, "code"=0, "source"=""} ("error out") -> [w533]
        tunnel: w150 -> [w526]
        shift-right: [w525] -> _
        shift-left: errorcluster {"status"=FALSE, "code"=0, "source"=""} ("error out") -> [w524]
        tunnel: w121 -> [w522]
        tunnel: w124 -> [w521]
        tunnel: w123 -> [w520]
        tunnel: w116 -> [w519]
        i -> [w518]
        stop <- w523 stop-if-true
        n177 = Greater Or Equal?(x=w518, y=100) -> (x >= y?=w515:bool)
        n178 = Get Queue Status(queue=w530, error in (no error)=w533) -> (queue out=w528:refnum<queue>, error out=w529:errorcluster, # elements in queue=w532:i32)  [unwired: 1 in, 5 out]
        n179 = Not Equal To 0?(x=w532) -> (x != 0?=w531:bool)
        n180 = And(x=w531, y=w515) -> (x .and. y?=w516:bool)
        n181 = case shown="True" w516 {
          tunnel: w529 -> [w535 w578]
          tunnel: w528 -> [_ w577]
          tunnel: [w535 w576] -> w527
          tunnel: w526 -> [_ w571]
          tunnel: [w534 w570] -> w525
          tunnel: w524 -> [w534 w569]
          tunnel: w522 -> [_ w566]
          tunnel: w521 -> [_ w565]
          tunnel: w520 -> [_ w564]
          tunnel: w519 -> [_ w554]
          frame False {
          }
          frame True {
            # "length"
            # "Waveform \nGenerator"
            n182 = Dequeue Element(queue=w577, error in (no error)=w578) -> (element=w538:i16[], error out=w576:errorcluster)  [unwired: 1 in, 2 out]
            n183 = Unbundle(w566) -> ("samples per symbol (16)"=w560:i32, "symbol map"=w553:cdb[])  [unwired: 1 out]
            n184 = Array Size(array=w538) -> (size(s)=w562:i32)
            n185 = Quotient & Remainder(x=w562, y=8) -> (floor(x/y)=w542:i32)  [unwired: 1 out]
            n186 = To Unsigned Word Integer(number=w542) -> (unsigned 16bit integer=w561:u16)
            n187 = Number To Boolean Array(number=w561) -> (Boolean array=w575:bool[])
            n188 = Reshape Array(w575, 2 ("dimension size"), 8 ("dimension size")) -> (w572:bool[][])
            n189 = for {
              tunnel: w572 -> [w581] mode=indexing
              tunnel: [w579] -> w563 mode=indexing
              n190 = Boolean Array To Number(Boolean array=w581) -> (number=w580:u32)
              n191 = To Unsigned Byte Integer(number=w580) -> (unsigned 8bit integer=w579:u8)
            }
            n192 = Initialize Array(u8 0, 128 ("dimension size")) -> (w537:u8[])
            n193 = Build Array (concatenate)(u8[] [53, 187, 37, 71, 79, 49, 4, 63] ("Array 2"), w563, w563) -> (w568:u8[])
            n194 = call "tx_pduGen.vi"("byte array"=w568) -> ("packet bits length"=→"packet bits length":i32, "pdu"=w539:i32[])  [unwired: 3 in]
            n195 = Build Array (concatenate)(w539, w538, w537) -> (w536:i32[])
            n196 = call "sub_bits_to_symbols.vi"("symbol map"=w553, "bits"=w536) -> ("symbols"=w552:cdb[])  [unwired: 9 in]
            n197 = Build Array (concatenate)(w552, w554) -> (w550:cdb[])
            n198 = call-poly <vilib>:"MT Pulse Shaping Filter.vi"("symbols"=w550, "pulse shaping filter coefficients"=w565, "samples per symbol (16)"=w560, "symbol rate (Hz)"=w564, "reset? (T)"=FALSE) -> ("output complex waveform"=w559:T10)  [unwired: 9 in, 1 out]
            n199 = Divide(x="Transmit power (db)", y=20.0) -> (x/y=w547:dbl)
            n200 = Unbundle(w559) -> ("t0"=w558:dbl, "dt"=w557:dbl, "Y"=w545:cdb[])
            n201 = Power Of 10(x=w547) -> (10^x=w546:dbl)
            n202 = Multiply(x=w545, y=w546) -> (x*y=w544:cdb[])
            n203 = Bundle(cluster=w559, "t0"=w558, "dt"=w557, "Y"=w544) -> (w556:T10)
            n204 = Enqueue Element(queue=w571, element=w556, error in (no error)=w569) -> (error out=w570:errorcluster)  [unwired: 1 in, 2 out]
          }
        }
        n205 = global read "var_stop.vi" "system stop"() -> (w523:bool)
      }
    }
    frame Error {
    }
  }
